vi "SPC_init_phot_stream.vi"(4 "#files_to_use":i16=-1 min=-1 max=999 step=1, 5 "fifo_type":T2 items=["48 bits SPC-6x0"=2, "32 bits SPC-6x0"=3, "32 bits SPC-130"=4, "32 bits SPC-830"=5, "32 bits SPC-140"=6, "32 bits SPC-150\\160\\180"=7, "32 bits DPC-230"=8, "32 bits FIFO_IMAGE"=9, "FIFO_D590"=10, "FIFO_TDC"=11, "FIFO_TDC_ABS"=12], 6 "stream_type":i16=1 max=1536 step=1 format="%x", 7 "spc_file":string="spcm_test.spc", 8 "Error In":errorcluster, 9 "what_to_read":T1, 10 "Modul No":i16, 11 "DLL Path":path) -> (0 "Error Out":errorcluster, 1 "Stream Handle":i16=-1, 2 "Modul No":i16, 3 "DLL Path":path)   [LabVIEW 2017]
doc: "fifo_type: 2 (FIFO_48), 3 (FIFO_32), 4 (FIFO_130), 5 (FIFO_830), 6 (FIFO_140), 7 (FIFO_150), 9 (FIFO_IMG)\n* spc_file file: path of the 1st spc file\nfiles_to_use: number of subsequent spc files to use, 1..999 or -1 for all files \nstream_type: bit 0 = 1- stream of BH .spc files ( 1st entry in each file contains MT clock, flags & rout.chan info)\n bit 0 = 0 - no special meaning of the first entry in the file\n bit 9 = 1 - stream contains marker entries ( FIFO_IMG mode )\n bit 10 = 1 - stream contains raw data ( diagnostics only )\nwhat_to_read: defines which entries will be extracted \n bit 0 = 1 read valid photons, bit 1 = 1 read invalid photons,\n bit 2 = 1 read markers 0 (pixel), bit 3 = 1 read markers 1 (line),\n bit 4 = 1 read markers 2 (frame), bit 5 = 1 read markers 3\n\nThe procedure is needed to initiate the process of extracting photons from a stream of .spc files created during FIFO measurement. \nIf the files were created using BH measurement software, 1st entry in each file contains Macro Time clock resolution and used routing channels information . In such case bit 0 of 'stream_type' parameter should be set to 1, otherwise if the 1st entry have no special meaning ( just photon frame) set it to 0. Set bit 9 of 'stream_type' if the file contains markers (was created in FIFO_IMG mode or FIFO mode with enabled markers).\nSubsequent files created in BH software during one measurement have 3 digits file number in file name part of the path ( for example xxx000.spc, xxx001.spc and so on). \nSuch files can be treated together during extracting photons ( they contain the same measurement) as a stream of files. \nWhen all photons from the 1st file will be extracted, the 2nd one will be opened during extraction and so on. The first file in the stream is given by 'spc_file' parameter and 'files_to_use' parameter tells how many files belong to the stream ( -1 means the procedure.will evaluate number of files in the stream and use it as 'files_to_use' value).\n'fifo_type parameter defines the format of the photons data in the stream. It depends mainly on the SPC module type which was used during the measurement. \nPossible 'fifo_type' values are defined in the spcm_def.h file.\n'what_to_read' parameter defines which entries will be extracted from the stream. \nIn most cases only bit 0 will be set ( valid photons ). For files containing also markers -\nmarkers 0-3 (pixel, line, frame) can also be extracted ( bits 2-5).\nIf the stream is successfully initialised, the procedure creates internal DLL PhotStreamInfo structure and returns the handle to the stream ( positive value). Use this handle as an input \nparameter to the other extraction functions ( SPC_close_phot_stream, SPC_get_phot_stream_info, SPC_get_photon).\nMax 8 streams can be initialised by the SPCM DLL.\nUse SPC_get_phot_stream_info to get the current state of the stream and SPC_get_photon to extract subsequent photons from the stream.\nAfter extracting photons stream should be closed using SPC_close_phot_stream function.\nSee use_spcm.c file for the extraction example. \n\ninfo@becker-hickl.com"
uses:
  SPC_Controls/Fifo_Type.ctl
  SPC_Controls/WhatToRead.ctl
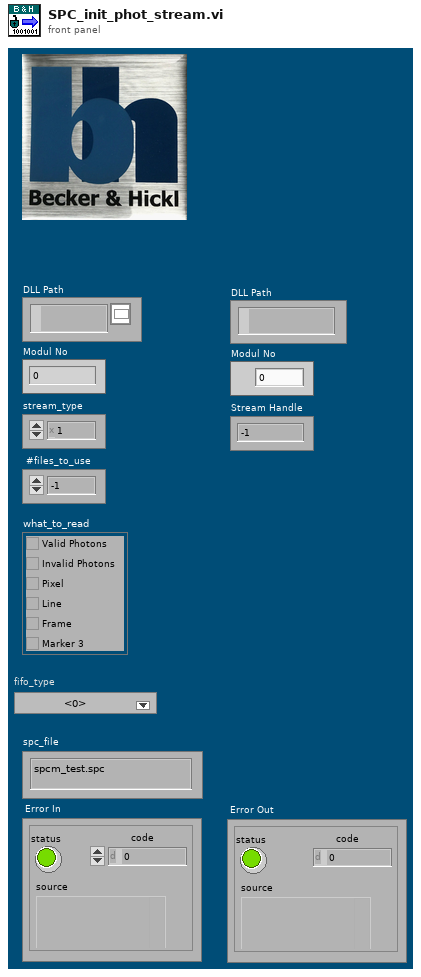
[diagram p1: front panel]
types:
  T1 = typedef "WhatToRead.ctl" = cluster{"Valid Photons":bool, "Invalid Photons":bool, "Pixel":bool, "Line":bool, "Frame":bool, "Marker 3":bool}
  T2 = typedef "Fifo_Type.ctl" = i16
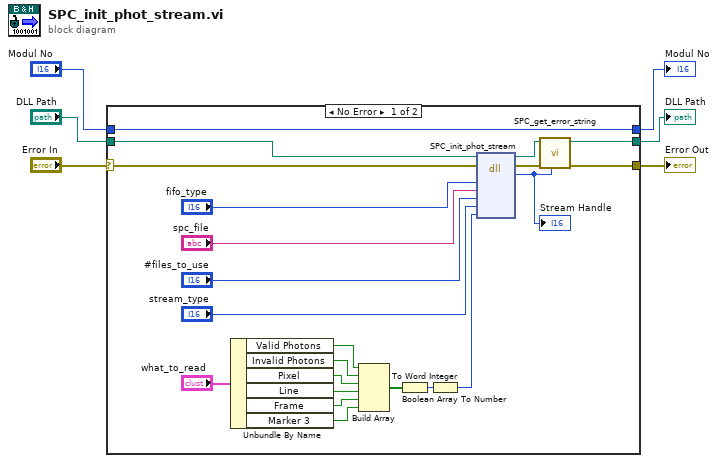
[diagram p0: block diagram]
diagram:
  n1 = case shown="No Error" "Error In" {
    selector: "Error In" -> [w24 w31]
    tunnel: [w20 w31] -> w5
    tunnel: "DLL Path" -> [w23 w30]
    tunnel: [w18 w30] -> w3
    tunnel: "Modul No" -> [w17 w29]
    tunnel: [w17 w29] -> w1
    frame No Error {
      n2 = Unbundle By Name("what_to_read") -> ("Valid Photons"=w15:bool, "Invalid Photons"=w14:bool, "Pixel"=w13:bool, "Line"=w12:bool, "Frame"=w11:bool, "Marker 3"=w10:bool)
      n3 = Build Array(w15, w14, w13, w12, w11, w10) -> (w9:bool[])
      n4 = Boolean Array To Number(Boolean array=w9) -> (number=w8:u32)
      n5 = To Word Integer(number=w8) -> (16bit integer=w7:i16)
      n6 = dll-call lib="D:/spcm/lib/lab_view/lv10.0/spcm32.dll" fn="SPC_init_phot_stream"(path in=w23, error in=w24, "fifo_type"="fifo_type", "spc_file"="spc_file", "files_to_use"="#files_to_use", "stream_type"="stream_type", "what_to_read"=w7) -> (path out=w19:path, error out=w21:errorcluster, "return type"=w22:i16)  [unwired: 6 in]
      "Stream Handle" <- w22
      n7 = call "SPC_get_error_string.vi"("ErrorID"=w22, "Error In"=w21, "DLL Path"=w19) -> ("Error Out"=w20:errorcluster, "DLL Path"=w18:path)  [unwired: 6 in, 1 out]
    }
    frame Error {
    }
  }
  "Error Out" <- w5
  "DLL Path" <- w3
  "Modul No" <- w1
